vi "ComponentSimulatorLauncher.vi"() -> ()   [LabVIEW 2018]
doc: "This vi launches the Component Simulator."
uses:
  src/TcpServer/configServerTypeDef.ctl
  src/TcpServerTel/typedef/enqueueOptionsTypeDef.ctl
  src/FactoryTcpServer/FactoryTcpServer.lvclass
  src/TcpServerTel/TcpServerTel.lvclass
  src/TcpServer/TcpServer.lvclass
panel:
  out "error out B":errorcluster
  out "error out A":errorcluster
  in  "error in (no error)":errorcluster
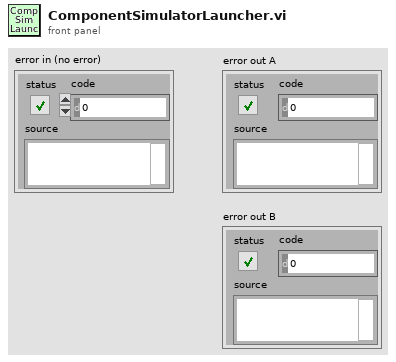
[diagram p1: front panel]
types:
  T1 = typedef "TcpServer.lvclass/configServerTypeDef.ctl" = cluster{"cmdServerPort":u16, "telServerPort":u16, "timeoutServerInMs":i32, "serverBytesToRead":i32, "maxSizeQueueTcpClientFromDds":i32, "EnqueueOptions":T2, "timeoutQueueTcpClientFromDds (ms)":i32, "maxSizeQueueTcpClient":i32, "timeoutInMs":i32}
  T2 = typedef "TcpServerTel.lvclass/enqueueOptionsTypeDef.ctl" = enum16{"lossy enqueue", "normal enqueue"}
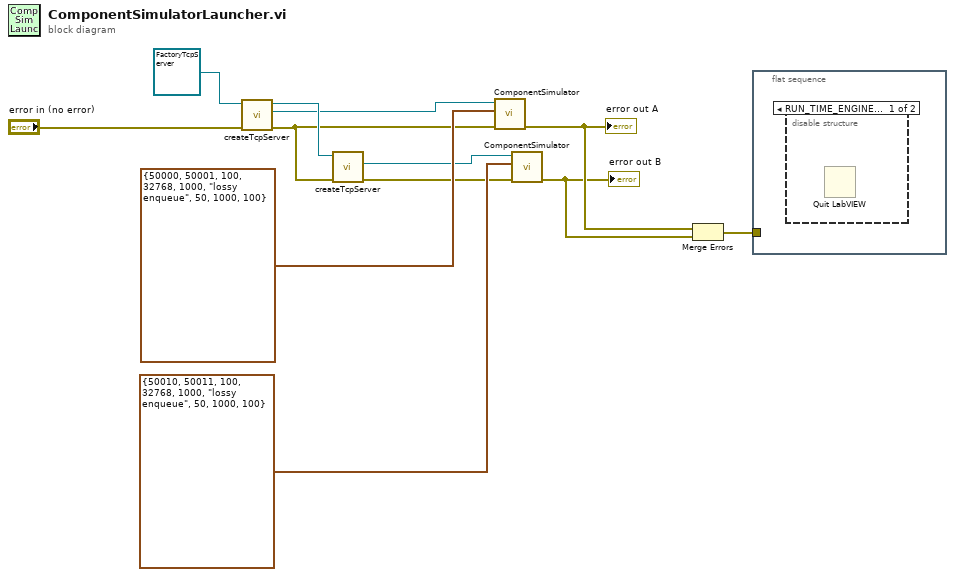
[diagram p0: block diagram]
diagram:
  n1 = call "createTcpServer.vi"("error in (no error)"="error in (no error)", "FactoryTcpServer in"=refnum<class "FactoryTcpServer.lvclass"> refnum ("FactoryTcpServer.lvclass")) -> ("error out"=w7:errorcluster, "TcpServer out"=w9:refnum<class "TcpServer.lvclass">, "FactoryTcpServer out"=w10:refnum<class "FactoryTcpServer.lvclass">)  [unwired: 7 in]
  n2 = call "createTcpServer.vi"("error in (no error)"=w7, "FactoryTcpServer in"=w10) -> ("error out"=w4:errorcluster, "TcpServer out"=w6:refnum<class "TcpServer.lvclass">)  [unwired: 7 in, 1 out]
  n3 = call "ComponentSimulator.vi"("error in"=w7, "ServerConfiguration"=T1 {"cmdServerPort"=50000, "telServerPort"=50001, "timeoutServerInMs"=100, "serverBytesToRead"=32768, "maxSizeQueueTcpClientFromDds"=1000, "EnqueueOptions"=enum."lossy enqueue", "timeoutQueueTcpClientFromDds (ms)"=50, "maxSizeQueueTcpClient"=1000, "timeoutInMs"=100}, "tcpServer in"=w9) -> ("error out"=w3:errorcluster)  [unwired: 8 in]
  "error out A" <- w3
  n4 = call "ComponentSimulator.vi"("error in"=w4, "ServerConfiguration"=T1 {"cmdServerPort"=50010, "telServerPort"=50011, "timeoutServerInMs"=100, "serverBytesToRead"=32768, "maxSizeQueueTcpClientFromDds"=1000, "EnqueueOptions"=enum."lossy enqueue", "timeoutQueueTcpClientFromDds (ms)"=50, "maxSizeQueueTcpClient"=1000, "timeoutInMs"=100}, "tcpServer in"=w6) -> ("error out"=w2:errorcluster)  [unwired: 8 in]
  "error out B" <- w2
  n5 = Merge Errors(w3, w2) -> (w1:errorcluster)
  n6 = flat-sequence {
    tunnel: w1 -> [_]
    frame #0 {
      n7 = disable-structure shown="RUN_TIME_ENGINE==True" {
        frame condition #0 {
          n8 = Quit LabVIEW() -> ()  [unwired: 1 in]
        }
        frame condition #1 (active) {
        }
      }
    }
  }
